vi "Result.Empty Str Data Check.vi"(7 "Code":i32=-4010, 10 "Data":string, 11 "Name":string) -> (2 "error out":errorcluster)   [LabVIEW 2019]
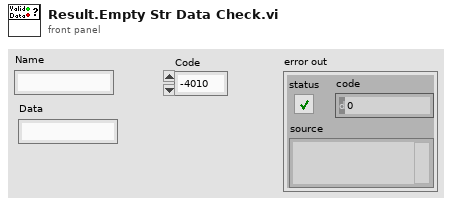
[diagram p1: front panel]
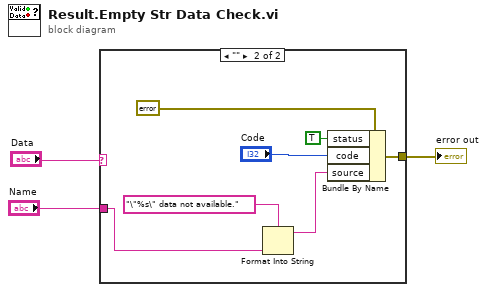
[diagram p0: block diagram]
diagram:
  n1 = case shown="\"\"" "Data" {
    tunnel: "Name" -> [_ w4]
    tunnel: [_ w7] -> w1
    frame "False", Default {
    }
    frame "" {
      n2 = Format Into String(format string="\"%s\" data not available." ("Category"), w4) -> (resulting string=w5:string)  [unwired: 2 in, 1 out]
      n3 = Bundle By Name(cluster=errorcluster {"status"=FALSE, "code"=0, "source"=""} ("error constant"), "status"=TRUE, "code"="Code", "source"=w5) -> (w7:errorcluster)
    }
  }
  "error out" <- w1
